vi "rqcAlice SPI.Set Delay Line Value.vi"(8 "error in":errorcluster, 10 "Delay Line Value":u32, 11 "Alice FPGA Reference In":refnum<k20>) -> (0 "error out":errorcluster, 3 "Alice FPGA Reference Out":refnum<k20>)   [LabVIEW 2019]
uses:
  Shared/Shared Host Lib/SPI/typedefs/SPI.FPGA Interface.ctl
  Shared/Shared Host Lib/SPI/typedefs/SPI.SubSystem.ctl
  <vilib>/Utility/error.llb/Error Cluster From Error Code.vi
  <vilib>/rvi/errors/niLvFpgaAdjustHostInterfaceError.vi
  <vilib>/rvi/interface/nirviReadWriteControl/nirviReadWriteControl.xnode
  NiFpgaLv.dll
  <vilib>/rvi/interface/Simulation/niFpgaSimulationCallBeginRW.vi
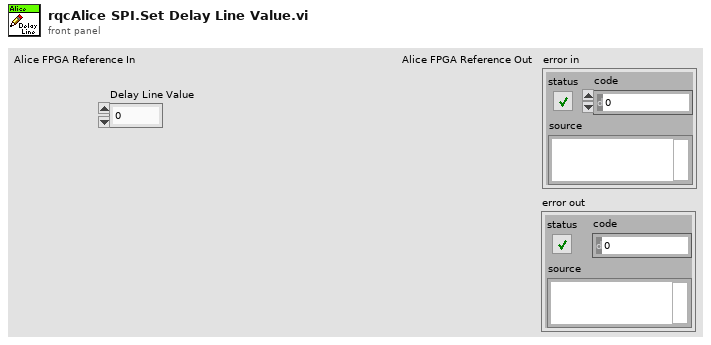
[diagram p1: front panel]
types:
  T1 = typedef "SPI.SubSystem.ctl" = enum8{"N/A", "DelayLine.MSB", "DelayLine.LSB", "Attenuation.dB", "Attenuation.DAC value", "SyncDetector.Offset", "SyncDetector.Comparator", "PM.Value[0]", "PM.Value[1]", "PM.Value[2]", "PM.Value[3]"}
  T2 = typedef "SPI.FPGA Interface.ctl" = refnum<k20>
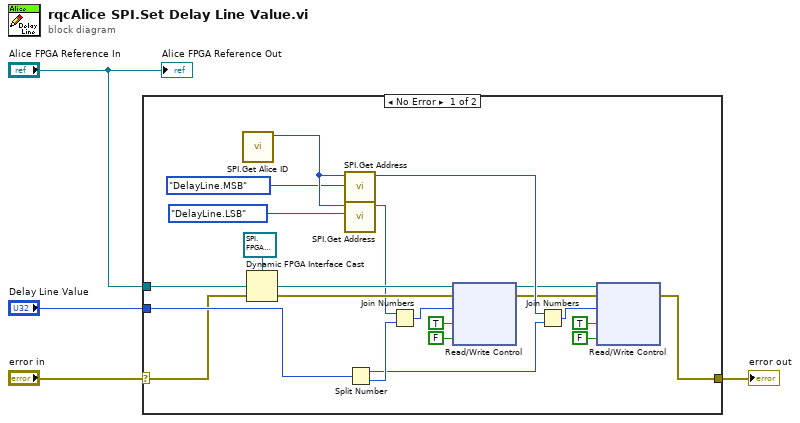
[diagram p0: block diagram]
diagram:
  n1 = case shown="No Error" "error in" {
    selector: "error in" -> [w12 w26]
    tunnel: [w21 w26] -> w3
    tunnel: "Alice FPGA Reference In" -> [w25 _]
    tunnel: "Delay Line Value" -> [w18 _]
    frame No Error {
      n2 = call "SPI.Get Alice ID.vi"() -> ("Alice.ID"=w11:u8)  [unwired: 11 in]
      n3 = Dynamic FPGA Interface Cast(Session In=T2 refnum ("Type"), Type=w25) -> (Session Out=w13:T2)
      n4 = call "SPI.Get Address.vi"("SPI.subSystem"=SPI.SubSystem."DelayLine.MSB", "ID"=w11) -> ("Address"=w9:u16)  [unwired: 9 in]
      n5 = call "SPI.Get Address.vi"("SPI.subSystem"=SPI.SubSystem."DelayLine.LSB", "ID"=w11) -> ("Address"=w10:u16)  [unwired: 9 in]
      n6 = Split Number(x=w18) -> (hi(x)=w14:u16, lo(x)=w15:u16)
      n7 = Join Numbers(hi=w10, lo=w15) -> ((hi.lo)=w16:u32)
      n8 = xnode "Read/Write Control"("FPGA VI Reference In"=w13, "error in"=w12, "SPI.data"=w16, "SPI.write"=TRUE ("reset"), "SPI.write"=FALSE ("reset")) -> ("FPGA VI Reference Out"=w8:T2, "error out"=w7:errorcluster)
      n9 = Join Numbers(hi=w9, lo=w14) -> ((hi.lo)=w17:u32)
      n10 = xnode "Read/Write Control"("FPGA VI Reference In"=w8, "error in"=w7, "SPI.data"=w17, "SPI.write"=TRUE, "SPI.write"=FALSE) -> ("error out"=w21:errorcluster)  [unwired: 1 out]
    }
    frame Error {
    }
  }
  "error out" <- w3
  "Alice FPGA Reference Out" <- "Alice FPGA Reference In"
